vi "CombinaisonSerrure.vi"() -> ()   [LabVIEW 2018]
panel:
  out "Numeric 4":u32
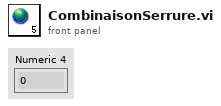
[diagram p1: front panel]
diagram:
